vi "FileReaderAuto.vi"(9 "index":i32, 11 "Auto Array":dbl[][](array[numeric]) format="%0.3f") -> (1 "Command ID":i16, 3 "Array":dbl[](array[numeric]))   [LabVIEW 2013]
panel:
  out "subarray 5":dbl[](array[numeric])
  out "subarray 4":dbl[](array[numeric])
  out "subarray 3":dbl[](array[numeric])
  out "subarray 2":dbl[](array[numeric])
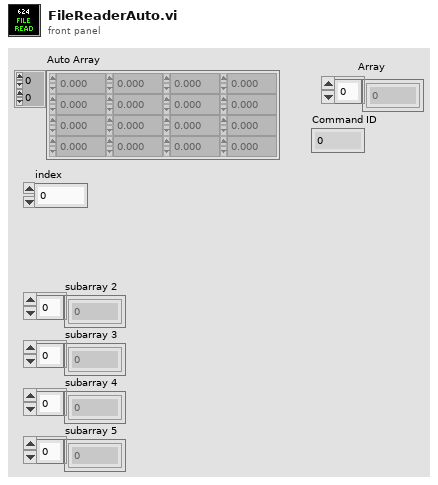
[diagram p1: front panel]
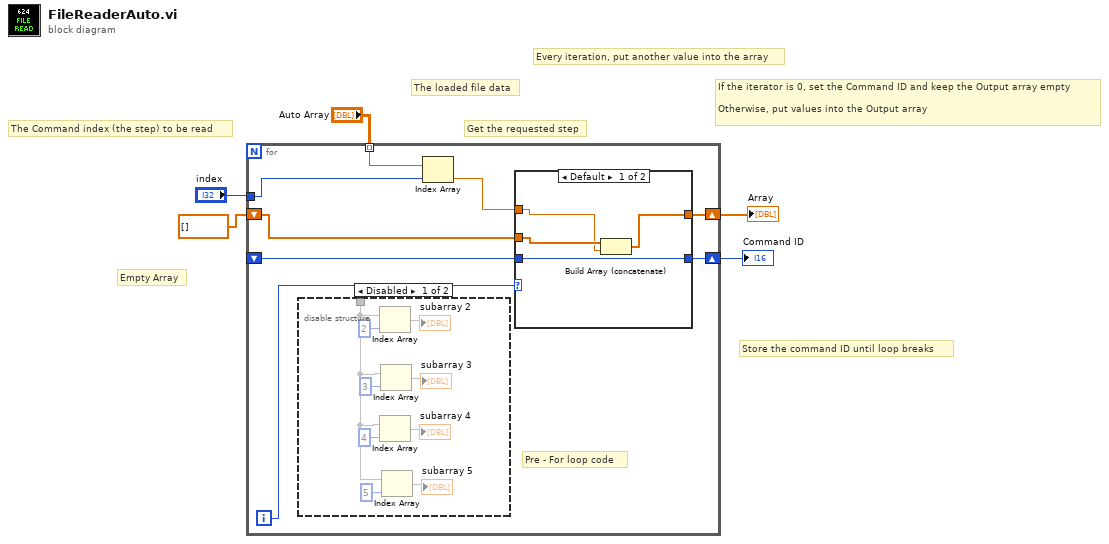
[diagram p0: block diagram]
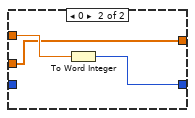
[diagram p2: hidden frame]
diagram:
  # "Store the command ID until loop breaks"
  # "Every iteration, put another value into the array"
  # "Empty Array"
  # "If the iterator is 0, set the Command ID and keep the Output array empty\n\nOtherwise, put values into the Output array"
  # "Get the requested step"
  # "The loaded file data"
  # "The Command index (the step) to be read"
  n1 = for {
    tunnel: "Auto Array" -> [w13] mode=indexing
    tunnel: "index" -> [w10]
    shift-right: [w9] -> w3
    shift-left: _ -> [w7]
    shift-right: [w8] -> w1
    shift-left: dbl[] [] ("Array") -> [w6]
    i -> [w12]
    # "Pre - For loop code"
    n2 = disable-structure shown="Disabled" {
      disable-tunnel: _ -> [w29 _]
      frame Disabled {
        n3 = Index Array(array=w29, index=2 ("index (row)")) -> (element=→"subarray 2")
        n4 = Index Array(array=w29, index=4 ("index (row)")) -> (element=→"subarray 4")
        n5 = Index Array(array=w29, index=3 ("index (row)")) -> (element=→"subarray 3")
        n6 = Index Array(array=w29, index=5 ("index (row)")) -> (element=→"subarray 5")
      }
      frame Enabled {
      }
    }
    n7 = Index Array(array=w13, index=w10) -> (element=w11:dbl)
    n8 = case shown="Default" w12 {
      tunnel: w11 -> [w15 w20]
      tunnel: [w17 w19] -> w9
      tunnel: [w14 w18] -> w8
      tunnel: w7 -> [w17 _]
      tunnel: w6 -> [w16 w18]
      frame Default {
        n9 = Build Array (concatenate)(w16, w15) -> (w14:dbl[])
      }
      frame 0 {
        n10 = To Word Integer(number=w20) -> (16bit integer=w19:i16)
      }
    }
  }
  "Array" <- w1
  "Command ID" <- w3
